vi "Find the Distance.vi"(11 "Relevant Data":T1[](array[typedef])) -> (3 "Distance":dbl)   [LabVIEW 2015]
uses:
  References/Relevant Data.ctl
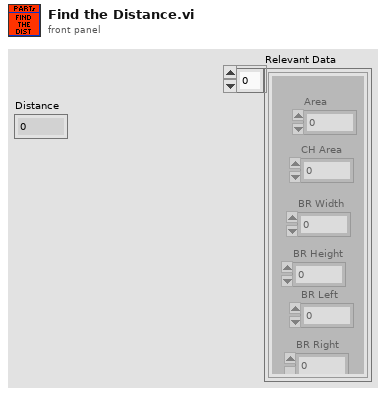
[diagram p1: front panel]
types:
  T1 = typedef "Relevant Data.ctl" = cluster{"Area":dbl, "CH Area":dbl, "BR Width":dbl, "BR Height":dbl, "BR Left":dbl, "BR Right":dbl}
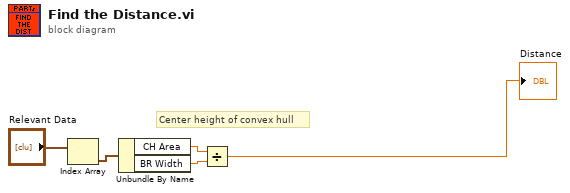
[diagram p0: block diagram]
diagram:
  # "Center height of convex hull"
  n1 = Index Array(array="Relevant Data") -> (element=w2:T1)  [unwired: 1 in]
  n2 = Unbundle By Name(w2) -> ("CH Area"=w4:dbl, "BR Width"=w5:dbl)
  n3 = Divide(x=w4, y=w5) -> (x/y=→"Distance":dbl)
